vi "SerialPort.Function_Connect.vi"(5 "Timeout(ms)":i32=4000, 7 "Module Name":string="Serial Port", 8 "error in":errorcluster, 11 "Q In":refnum<queue>) -> (0 "error out":errorcluster)   [LabVIEW 2018]
uses:
  <vilib>/KATE/Queues/Q.Element.ctl
  <vilib>/KATE/Queues/Queue Utils.lvlib
panel:
  # "Serial Port Connect"
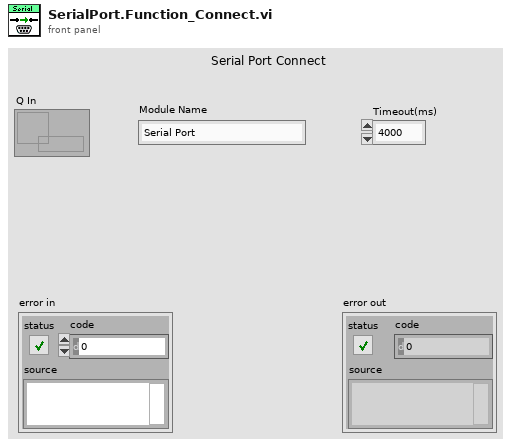
[diagram p1: front panel]
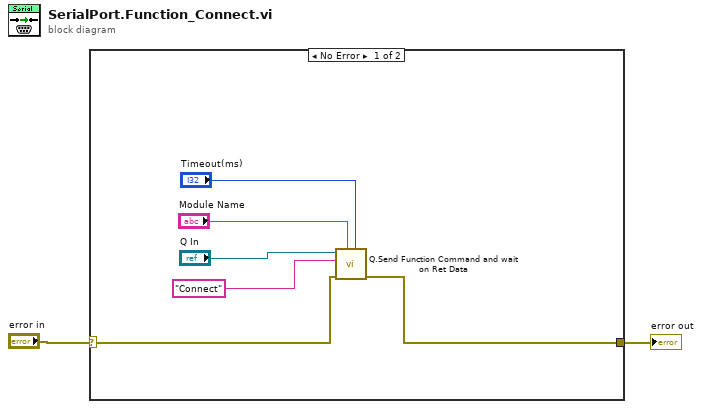
[diagram p0: block diagram]
diagram:
  n1 = case shown="No Error" "error in" {
    selector: "error in" -> [w4 w9]
    tunnel: [w3 w9] -> w1
    frame No Error {
      n2 = call <vilib>:"Q.Send Function Command and wait on Ret Data.vi"("Timeout(ms)"="Timeout(ms)", "Q Name"="Module Name", "error in"=w4, "Cmd"="Connect", "Q In"="Q In") -> ("error out"=w3:errorcluster)  [unwired: 5 in, 1 out]
    }
    frame Error {
    }
  }
  "error out" <- w1
